vi "count channels.vi"(11 "Array":bool[](array[boolean])) -> (3 "Chan 3":i16)   [LabVIEW 2024]
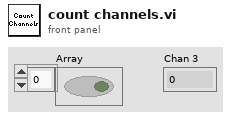
[diagram p1: front panel]
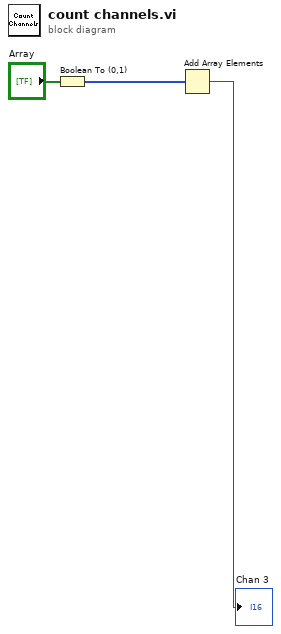
[diagram p0: block diagram]
diagram:
  n1 = Boolean To (0,1)(Boolean="Array") -> (0, 1=w2:i16[])
  n2 = Add Array Elements(numeric array=w2) -> (sum=→"Chan 3":i16)
